vi "Write 2D History Array to NT Table.vi"(11 "History Data":dbl[][](array[numeric])) -> ()   [LabVIEW 2016]
uses:
  <vilib>/Rock Robotics/Network Tables/NT Write String.vi
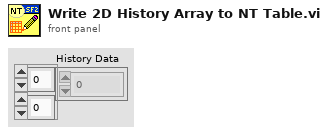
[diagram p1: front panel]
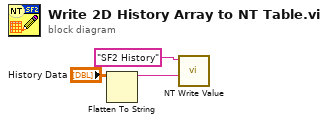
[diagram p0: block diagram]
diagram:
  n1 = Flatten To String(anything="History Data") -> (data string=w1:string)  [unwired: 3 in, 2 out]
  n2 = call-poly <vilib>:"NT Write Value.vi"("String"=w1, "Name"="SF2 History") -> ()  [unwired: 9 in, 1 out]
